vi "Flatten.vi"(8 "error in":errorcluster, 9 "Data":T1) -> (0 "error out":errorcluster, 2 "Buffer":u8[](array[numeric]) format="%.0x")   [LabVIEW 2020, in "Event.lvlib"]
uses:
  Event.lvlib
  Data.ctl
  lv-protoc/LV-Proto/LV-Proto.lvlib
  EventLevel/EventLevel.lvlib
  Error/Error.lvlib
  EventLevel/Enumeration.ctl
  Error/Data.ctl
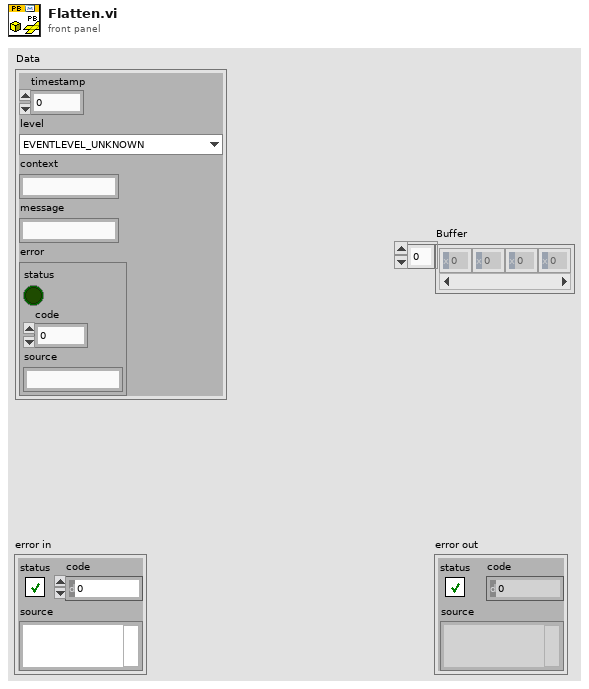
[diagram p1: front panel]
types:
  T1 = typedef "Event.lvlib/Data.ctl" = cluster{"timestamp":i64, "level":T2, "context":string, "message":string, "error":T3}
  T2 = typedef "EventLevel.lvlib/Enumeration.ctl" = enum16{"EVENTLEVEL_UNKNOWN", "EVENTLEVEL_DEBUG", "EVENTLEVEL_INFO", "EVENTLEVEL_WARNING", "EVENTLEVEL_ERROR"}
  T3 = typedef "Error.lvlib/Data.ctl" = errorcluster
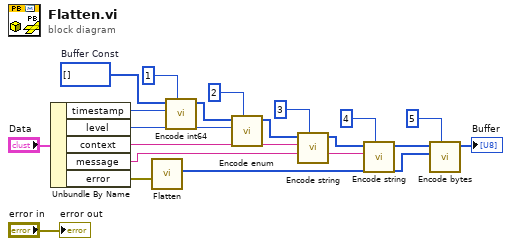
[diagram p0: block diagram]
diagram:
  w17 = u8[] []  # Buffer Const
  n1 = Unbundle By Name("Data") -> ("timestamp"=w15:i64, "level"=w12:T2, "context"=w9:string, "message"=w6:string, "error"=w5:T3)
  n2 = call "Flatten.vi"("Data"=w5) -> ("Buffer"=w3:u8[])  [unwired: 9 in, 1 out]
  n3 = call "Encode int64.vi"("Field Number"=1, "int64"=w15, "Buffer in"=w17) -> ("Buffer"=w14:u8[])  [unwired: 8 in]
  n4 = call "Encode enum.vi"("Field Number"=2, "Enumeration"=w12, "Buffer in"=w14) -> ("Buffer"=w11:u8[])  [unwired: 8 in]
  n5 = call "Encode string.vi"("Field Number"=3, "string"=w9, "Buffer in"=w11) -> ("Buffer"=w8:u8[])  [unwired: 8 in]
  n6 = call "Encode string.vi"("Field Number"=4, "string"=w6, "Buffer in"=w8) -> ("Buffer"=w4:u8[])  [unwired: 8 in]
  n7 = call "Encode bytes.vi"("Field Number"=5, "bytes"=w3, "Buffer in"=w4) -> ("Buffer"=→"Buffer":u8[])  [unwired: 8 in]
  "error out" <- "error in"
